vi "overflow_control_alu.vi"(1 "CONTROL":T1, 2 "over_divide":bool, 3 "over_multiply":bool, 4 "over_sum":bool) -> (0 "over_flag":bool)   [LabVIEW 2013]
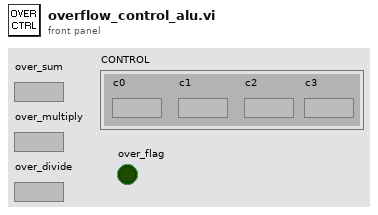
[diagram p1: front panel]
types:
  T1 = cluster{"c0":bool, "c1":bool, "c2":bool, "c3":bool}
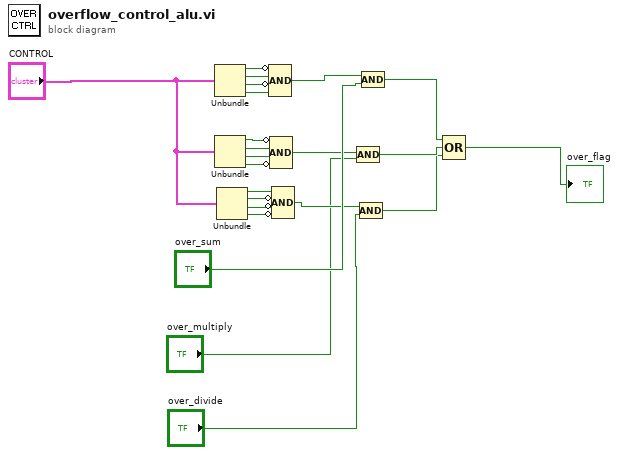
[diagram p0: block diagram]
diagram:
  n1 = Unbundle("CONTROL") -> ("c0"=w23:bool, "c1"=w22:bool, "c2"=w21:bool, "c3"=w20:bool)
  n2 = Unbundle("CONTROL") -> ("c0"=w19:bool, "c1"=w18:bool, "c2"=w17:bool, "c3"=w16:bool)
  n3 = Unbundle("CONTROL") -> ("c0"=w14:bool, "c1"=w13:bool, "c2"=w12:bool, "c3"=w11:bool)
  n4 = Compound Arithmetic op=AND(invert w23, w22, invert w21, w20) -> (w9:bool)
  n5 = Compound Arithmetic op=AND(invert w19, w18, w17, invert w16) -> (w8:bool)
  n6 = Compound Arithmetic op=AND(w14, invert w13, invert w12, invert w11) -> (w7:bool)
  n7 = Compound Arithmetic op=AND(w8, "over_multiply") -> (w3:bool)
  n8 = Compound Arithmetic op=AND(w7, "over_divide") -> (w2:bool)
  n9 = Compound Arithmetic op=AND(w9, "over_sum") -> (w4:bool)
  n10 = Compound Arithmetic op=OR(w4, w3, w2) -> (→"over_flag":bool)
